vi "testGetNonOverlapIdx.vi"(8 "error in (no error)":errorcluster) -> (0 "error out":errorcluster)   [LabVIEW 2016]
doc: "Test to get the non overlap index array from the input index array."
uses:
  <vilib>/addons/_JKI Toolkits/Caraya/classes/Assert/Assert.lvclass
  <vilib>/addons/_JKI Toolkits/Caraya/classes/Test/Test.lvclass
  MatOper/MatOper.lvclass
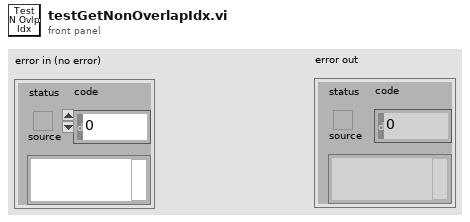
[diagram p1: front panel]
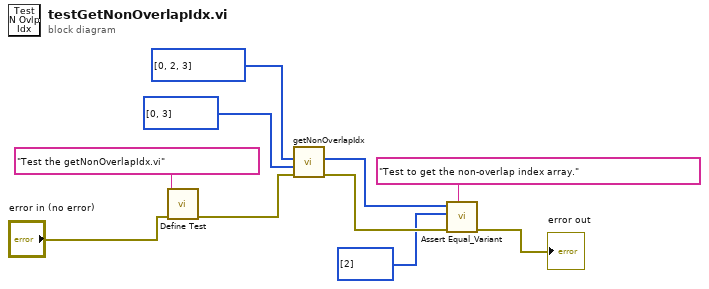
[diagram p0: block diagram]
diagram:
  n1 = call <vilib>:"Define Test.vi"("error in (no error)"="error in (no error)", "Label (VI Title)"="Test the getNonOverlapIdx.vi") -> ("error out"=w6:errorcluster)  [unwired: 9 in]
  n2 = call "getNonOverlapIdx.vi"("error in (no error)"=w6, "Overlap Idx Array"=i32[] [0, 3], "Input Idx Array"=i32[] [0, 2, 3]) -> ("error out"=w5:errorcluster, "Non-Overlap Idx Array"=w4:i32[])  [unwired: 6 in, 1 out]
  n3 = call <vilib>:"Assert Equal_Variant.vi"("Label"="Test to get the non-overlap index array.", "error in (no error)"=w5, "Y"=i32[] [2] ("Non-Overlap Idx Array"), "X"=w4) -> ("error out"=→"error out":errorcluster)  [unwired: 7 in]
